vi "Teleop_System_Acquire_Decide.vi"(8 "error in (no error)":errorcluster) -> (0 "error out":errorcluster)   [LabVIEW 2019]
uses:
  <vilib>/Rock Robotics/WPI/ThirdParty/JAS_Junk/TrajLib/Rotation2d_CreateAngleDegrees.vi
  <vilib>/Rock Robotics/WPI/ThirdParty/JAS_Junk/TrajLib/Conv_Deg_Radians.vi
  <vilib>/Rock Robotics/WPI/ThirdParty/JAS_Junk/TrajLib/Rotation2d_CreateAngle.vi
  <vilib>/Rock Robotics/WPI/Utilities/WPI_GetSetVariantRefNum.vi
  Teleop_System_Globals.vi
  <vilib>/Rock Robotics/WPI/Joystick/WPI_JoystickArcadeMapping.vi
  Diff_Drive_System/Diff_Drive_System_Globals.vi
  Trajectory_Execution_Diff_Drive/Trajectory_Execution_Globals.vi
  <vilib>/Rock Robotics/WPI/ThirdParty/JAS_Junk/TrajLib/Trajectory_Library.lvlib
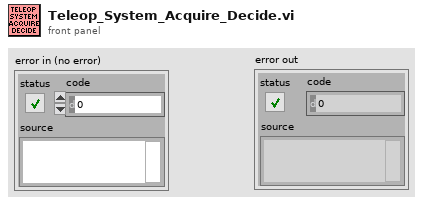
[diagram p1: front panel]
types:
  T1 = typedef "WPI_JoystickDevRef.ctl" = cluster{"Device":T2}
  T2 = typedef "WPI_JoystickDeviceEnum.ctl" = enum16{"USB 0", "USB 1", "USB 2", "USB 3", "USB 4", "USB 5"}
  T3 = typedef "Trajectory_Execution_Sensors.ctl" = cluster{"Left Distance":dbl, "Right Distance":dbl, "Gyro Continous\n (inc counterclockwise)":dbl, "Left Speed":dbl, "Right Speed":dbl}
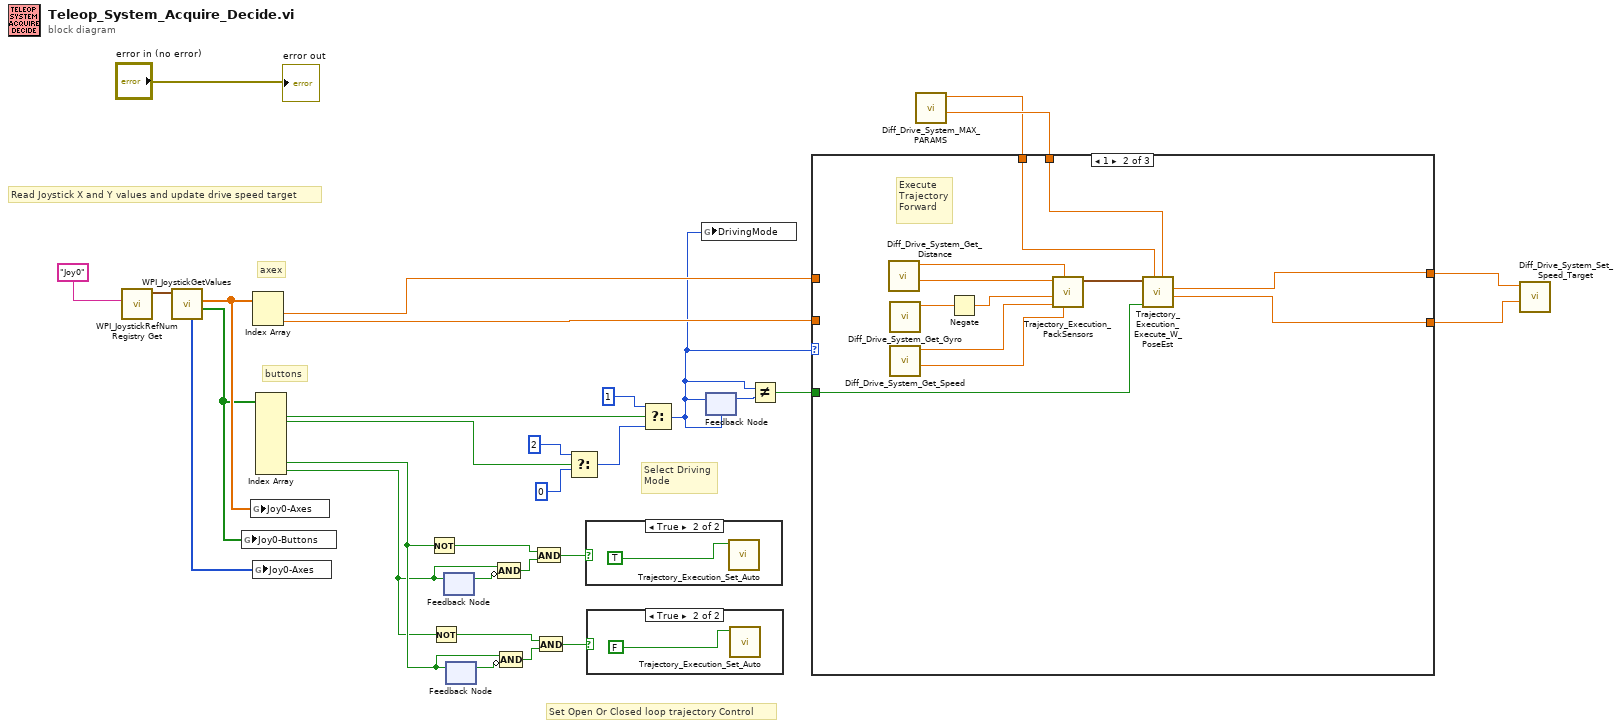
[diagram p0: block diagram]
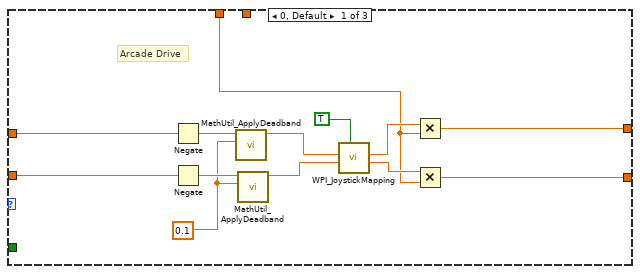
[diagram p4: hidden frame]
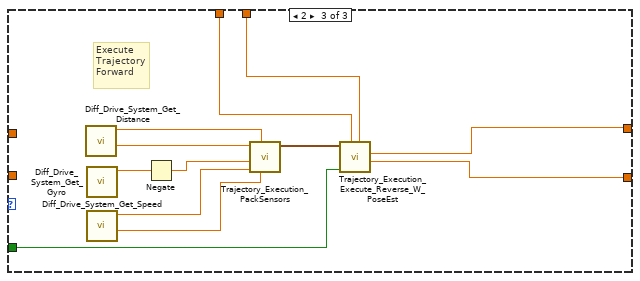
[diagram p5: hidden frame]
diagram:
  # "Set Open Or Closed loop trajectory Control"
  # "Select Driving\nMode"
  # "buttons"
  # "axex"
  # "Read Joystick X and Y values and update drive speed target"
  n1 = call <vilib>:"WPI_JoystickRefNum Registry Get.vi"("refnum name"="Joy0") -> ("JoystickDevRef"=w9:T1)  [unwired: 1 in, 9 out]
  n2 = call <vilib>:"WPI_JoystickGetValues.vi"("JoystickDevRef"=w9) -> ("Buttons"=w6:bool[], "Axes"=w7:dbl[], "POVs"=w5:i16[])  [unwired: 6 in, 2 out]
  n3 = global write "Teleop_System_Globals.vi" "Joy0-Buttons"(w6) -> ()
  n4 = global write "Teleop_System_Globals.vi" "Joy0-Axes"(w7) -> ()
  n5 = Index Array(array=w7) -> (element #1=w10:dbl, element #2=w11:dbl)  [unwired: 2 in]
  n6 = global write "Teleop_System_Globals.vi" "Joy0-Axes"(w5) -> ()
  n7 = Index Array(array=w6) -> (element #1=w14:bool, element #2=w20:bool, element #7=w31:bool, element #8=w30:bool)  [unwired: 8 in, 4 out]
  n8 = Not(x=w31) -> (.not. x?=w24:bool)
  n9 = Not(x=w30) -> (.not. x?=w27:bool)
  n10 = feedback #1() -> (w22:bool)  [unwired: 1 in]
  n11 = feedback-in #1(w30) -> ()
  n12 = feedback #2() -> (w25:bool)  [unwired: 1 in]
  n13 = feedback-in #2(w31) -> ()
  n14 = Compound Arithmetic op=AND(w30, invert w22) -> (w23:bool)
  n15 = Compound Arithmetic op=AND(w31, invert w25) -> (w26:bool)
  n16 = And(x=w24, y=w23) -> (x .and. y?=w29:bool)
  n17 = And(x=w27, y=w26) -> (x .and. y?=w28:bool)
  n18 = Select(t=2, s=w20, f=0) -> (s? t:f=w19:i32)
  n19 = case shown="True" w29 {
    frame False {
    }
    frame True {
      n20 = call "Trajectory_Execution_Set_Auto.vi"("Ramsete AUTO"=TRUE ("Traj_RamseteEnabled")) -> ()  [unwired: 11 in]
    }
  }
  n21 = case shown="True" w28 {
    frame False {
    }
    frame True {
      n22 = call "Trajectory_Execution_Set_Auto.vi"("Ramsete AUTO"=FALSE ("Traj_RamseteEnabled")) -> ()  [unwired: 11 in]
    }
  }
  n23 = Select(t=1, s=w14, f=w19) -> (s? t:f=w1:i32)
  n24 = global write "Teleop_System_Globals.vi" "DrivingMode"(w1) -> ()
  n25 = feedback #3(w1) -> (w15:i32)
  n26 = feedback-in #3(w1) -> ()
  n27 = Not Equal?(x=w1, y=w15) -> (x != y?=w16:bool)
  n28 = call "Diff_Drive_System_MAX_PARAMS.vi"() -> ("Effective TrackWidth Ft"=w21:dbl, "Max Speed Ft/Sec"=w12:dbl)  [unwired: 10 in]
  n29 = case shown="1" w1 {
    tunnel: w10 -> [w45 _ _]
    tunnel: w11 -> [w44 _ _]
    tunnel: [w43 w56 w60] -> w3
    tunnel: [w42 w55 w59] -> w2
    tunnel: w12 -> [w39 w57 w62]
    tunnel: w16 -> [_ w58 w61]
    tunnel: w21 -> [_ w54 w63]
    frame 0, Default {
      w34 = 0.1 ("Deadband")
      # "Arcade Drive"
      n30 = Negate(x=w45) -> (-x=w37:dbl)
      n31 = Negate(x=w44) -> (-x=w36:dbl)
      n32 = call <vilib>:"MathUtil_ApplyDeadband.vi"("Deadband"=w34, "Value"=w37) -> ("Result"=w38:dbl)  [unwired: 9 in]
      n33 = call <vilib>:"MathUtil_ApplyDeadband.vi"("Deadband"=w34, "Value"=w36) -> ("Result"=w35:dbl)  [unwired: 9 in]
      n34 = call-poly <vilib>:"WPI_JoystickMapping.vi"("Square Inputs"=TRUE, "Y axis value"=w35, "X axis value"=w38) -> ("Right Motor Value"=w40:dbl, "Left Motor Value"=w41:dbl)  [unwired: 7 in]
      n35 = Multiply(x=w41, y=w39) -> (x*y=w43:dbl)
      n36 = Multiply(x=w40, y=w39) -> (x*y=w42:dbl)
    }
    frame 1 {
      # "Execute\nTrajectory\nForward"
      n37 = call "Diff_Drive_System_Get_Distance.vi"() -> ("Right Distance FT"=w50:dbl, "Left Distance FT"=w51:dbl)  [unwired: 10 in]
      n38 = call "Diff_Drive_System_Get_Gyro.vi"() -> ("Gyro_DEG"=w53:dbl)  [unwired: 10 in, 1 out]
      n39 = call "Diff_Drive_System_Get_Speed.vi"() -> ("Right Speed FT/S"=w47:dbl, "Left Speed FT/S"=w48:dbl)  [unwired: 10 in]
      n40 = Negate(x=w53) -> (-x=w49:dbl)
      n41 = call "Trajectory_Execution_PackSensors.vi"("Right Speed"=w47, "Left Distance"=w51, "Left Speed"=w48, "Gyro Continous\n (inc counterclockwise)"=w49, "Right Distance"=w50) -> ("Input Sensors"=w52:T3)  [unwired: 6 in]
      n42 = call "Trajectory_Execution_Execute_W_PoseEst.vi"("Effective Track Width FT"=w54, "Max Speed\nFT/SEC"=w57, "Init"=w58, "Input Sensors"=w52) -> ("Right Speed Target"=w55:dbl, "Left Speed Target"=w56:dbl)  [unwired: 3 in, 3 out]
    }
    frame 2 {
      # "Execute\nTrajectory\nForward"
      n43 = call "Diff_Drive_System_Get_Distance.vi"() -> ("Right Distance FT"=w67:dbl, "Left Distance FT"=w68:dbl)  [unwired: 10 in]
      n44 = call "Diff_Drive_System_Get_Gyro.vi"() -> ("Gyro_DEG"=w70:dbl)  [unwired: 10 in, 1 out]
      n45 = call "Diff_Drive_System_Get_Speed.vi"() -> ("Right Speed FT/S"=w64:dbl, "Left Speed FT/S"=w65:dbl)  [unwired: 10 in]
      n46 = Negate(x=w70) -> (-x=w66:dbl)
      n47 = call "Trajectory_Execution_PackSensors.vi"("Right Speed"=w64, "Left Distance"=w68, "Left Speed"=w65, "Gyro Continous\n (inc counterclockwise)"=w66, "Right Distance"=w67) -> ("Input Sensors"=w69:T3)  [unwired: 6 in]
      n48 = call "Trajectory_Execution_Execute_Reverse_W_PoseEst.vi"("Effective Track Width FT"=w63, "Max Speed\nFT/SEC"=w62, "Init"=w61, "Input Sensors"=w69) -> ("Right Speed Target"=w59:dbl, "Left Speed Target"=w60:dbl)  [unwired: 3 in, 3 out]
    }
  }
  n49 = call "Diff_Drive_System_Set_Speed_Target.vi"("Right Speed Target FT/S"=w2, "Left Speed Target FT/S"=w3) -> ()  [unwired: 10 in]
  "error out" <- "error in (no error)"
